vi "SEA_9811_VS_Write.vi"(8 "error in (no error)":errorcluster, 11 "SEA9811_RT_data in":T1 {"Tx"."Tx Refs (Data,Trig)"."Data Reference" format="%.0x"}) -> (0 "error out":errorcluster, 3 "SEA9811_RT_data out":T1 {"Tx"."Tx Refs (Data,Trig)"."Data Reference" format="%.0x"})   [LabVIEW 2015]
uses:
  Typdefs/SEA9811_RT_data_cluster.ctl
  <userlib>/_FPGA Interface Advanced Tools/FPGA Interface Base/FPGA Interface Base.lvclass
  Typdefs/FPGA ref.ctl
  Typdefs/channel.ctl
  Typdefs/received word.ctl
  Typdefs/SEA9811_FPGA_FP_Addresses.ctl
  <vilib>/NI Veristand/Custom Device API/Block Data Reference.ctl
  <vilib>/NI Veristand/Custom Device API/Data Reference.ctl
  <userlib>/_FPGA Interface Advanced Tools/FPGA Interface Wrapper/NiFPGA Write - U32.vi
  <userlib>/_FPGA Interface Advanced Tools/FPGA Interface Wrapper/NiFPGA Write - Boolean.vi
  <vilib>/NI Veristand/Custom Device API/Global Data Refs.vi
  <vilib>/Utility/error.llb/Error Cluster From Error Code.vi
  <userlib>/_FPGA Interface Advanced Tools/FPGA Interface Wrapper/FPGA Interface Wrapper.lvlib
  <vilib>/NI VeriStand/Custom Device API/Custom Device API.lvlib
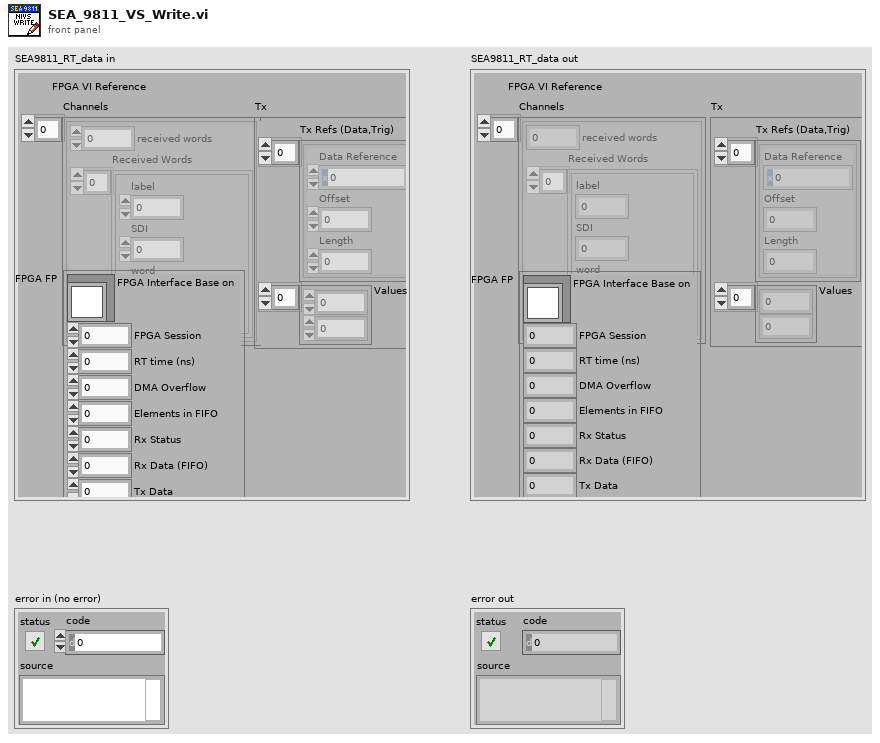
[diagram p1: front panel]
types:
  T1 = typedef "SEA9811_RT_data_cluster.ctl" = cluster{"FPGA VI Reference":T2, "Channels":T3[], "FPGA FP":T5, "Tx":cluster{"Tx Refs (Data,Trig)":T6[], "Values":dbl[]}}
  T2 = typedef "FPGA ref.ctl" = refnum<k20>
  T3 = typedef "channel.ctl" = cluster{"received words":u32, "Received Words":T4[]}
  T4 = typedef "received word.ctl" = cluster{"label":u8, "SDI":u8, "word":u32, "timestamp":dbl}
  T5 = typedef "SEA9811_FPGA_FP_Addresses.ctl" = cluster{"FPGA Interface Base on":refnum<class "FPGA Interface Base.lvclass">, "FPGA Session":u32, "RT time (ns)":u32, "DMA Overflow":u32, "Elements in FIFO":u32, "Rx Status":u32, "Rx Data (FIFO)":u32, "Tx Data":u32, "Transmit Data":u32}
  T6 = typedef "Custom Device API.lvlib/Block Data Reference.ctl" = cluster{"Data Reference":T7, "Offset":u64, "Length":u64}
  T7 = typedef "Custom Device API.lvlib/Data Reference.ctl" = i32
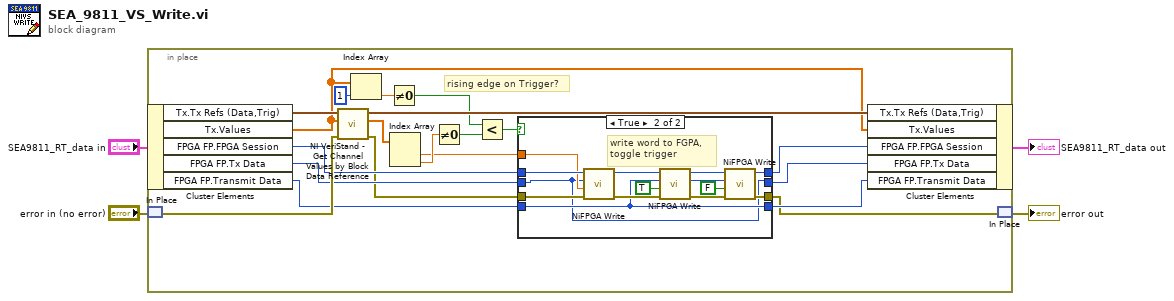
[diagram p0: block diagram]
diagram:
  n1 = in-place {
    # "rising edge on Trigger?"
    n2 = in-place-cluster #1("SEA9811_RT_data in") -> ("Tx.Tx Refs (Data,Trig)"=w24:T6[], "Tx.Values"=w9:dbl[], "FPGA FP.FPGA Session"=w14:u32, "FPGA FP.Tx Data"=w13:u32, "FPGA FP.Transmit Data"=w10:u32)
    n3 = in-place-match #2("error in (no error)") -> (w23:errorcluster)
    n4 = call <vilib>:"NI VeriStand - Get Channel Values by Block Data Reference.vi"("error in (no error)"=w23, "Values Array in"=w9, "Block Data Ref"=w24) -> ("error out"=w12:errorcluster, "Values Array out"=w20:dbl[], "Block Data Ref dup"=w22:T6[])  [unwired: 6 in]
    n5 = Index Array(array=w9, index=1) -> (element=w19:dbl)
    n6 = Not Equal To 0?(x=w19) -> (x != 0?=w17:bool)
    n7 = Index Array(array=w20) -> (element #1=w11:dbl, element #2=w18:dbl)  [unwired: 2 in]
    n8 = Not Equal To 0?(x=w18) -> (x != 0?=w16:bool)
    n9 = Less?(x=w17, y=w16) -> (x < y?=w15:bool)
    n10 = case shown="True" w15 {
      tunnel: w14 -> [w28 w41]
      tunnel: w13 -> [w27 w29]
      tunnel: w12 -> [w25 w40]
      tunnel: w11 -> [_ w39]
      tunnel: w10 -> [w26 w30]
      tunnel: [w25 w32] -> w5
      tunnel: [w28 w31] -> w8
      tunnel: [w27 w29] -> w7
      tunnel: [w26 w30] -> w6
      frame False {
      }
      frame True {
        # "write word to FGPA,\ntoggle trigger"
        # "one of the values changed"
        n11 = call-poly <userlib>:"NiFPGA Write.vi"("error in (no error)"=w40, "Value"=w39, "Control"=w29, "Session"=w41) -> ("error out"=w37:errorcluster, "Session Out"=w38:u32)  [unwired: 6 in]
        n12 = call-poly <userlib>:"NiFPGA Write.vi"("error in (no error)"=w37, "Boolean"=TRUE, "Control"=w30, "Session"=w38) -> ("error out"=w33:errorcluster, "Session Out"=w34:u32)  [unwired: 6 in]
        n13 = call-poly <userlib>:"NiFPGA Write.vi"("error in (no error)"=w33, "Boolean"=FALSE, "Control"=w30, "Session"=w34) -> ("error out"=w32:errorcluster, "Session Out"=w31:u32)  [unwired: 6 in]
      }
    }
    n14 = in-place-cluster #1("Tx.Tx Refs (Data,Trig)"=w22, "Tx.Values"=w9, "FPGA FP.FPGA Session"=w8, "FPGA FP.Tx Data"=w7, "FPGA FP.Transmit Data"=w6) -> (→"SEA9811_RT_data out":T1)
    n15 = in-place-match #2(w5) -> (→"error out":errorcluster)
  }
